vi "Draw.vi"(5 "Angle":dbl, 6 "Scale":sgl=1.0, 7 "Rotation Center":refnum<class "Vector 2D.lvclass">, 8 "error in (no error)":errorcluster, 9 "Destination":refnum<class "Vector 2D.lvclass">, 10 "Texture":refnum<class "Texture.lvclass">, 11 "Renderer":refnum<class "Renderer.lvclass">) -> (0 "error out":errorcluster)   [LabVIEW 2021, in "Renderer.lvclass"]
uses:
  Renderer.lvclass
  Texture/Texture.lvclass
  Vector 2D/Vector 2D.lvclass
  Renderer.lvclass/Renderer.ctl
  LabSDL2/Source/Libraries/LibSDL2 Wrapper/Controls/NULL.ctl
  LabSDL2/Source/Libraries/LibSDL2 Wrapper/LibSDL2.lvlib
  LabSDL2/Source/Libraries/LibSDL2 Wrapper/Controls/Rectangle.ctl
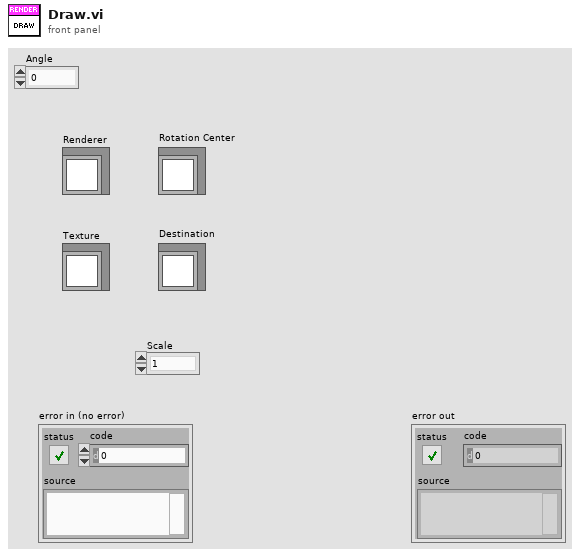
[diagram p1: front panel]
types:
  T1 = typedef "LibSDL2.lvlib/NULL.ctl" = enum32{"NULL"}
  T2 = typedef "LibSDL2.lvlib/Rectangle.ctl" = cluster{"x":i32, "y":i32, "Width":i32, "Height":i32}
  T3 = typedef "SDL2 Utility.lvlib/Point (I32).ctl" = cluster{"x":i32, "y":i32}
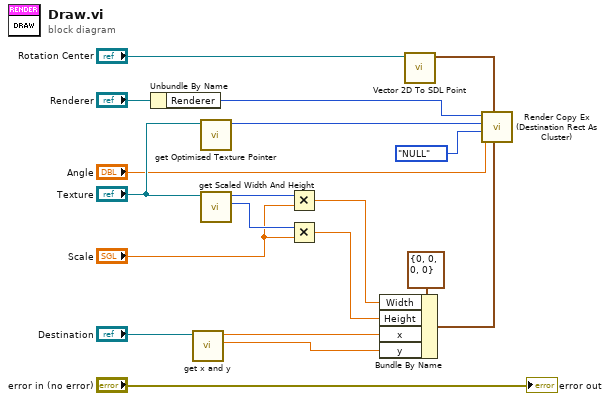
[diagram p0: block diagram]
diagram:
  n1 = Unbundle By Name("Renderer") -> ("Renderer"=w15:u32)
  n2 = call "get x and y.vi"("Vector 2D in"="Destination") -> ("y"=w5:sgl, "x"=w6:sgl)  [unwired: 9 in]
  n3 = call "get Optimised Texture Pointer.vi"("Texture in"="Texture") -> ("Optimised Texture Pointer"=w16:u32)  [unwired: 10 in]
  n4 = call "get Scaled Width And Height.vi"("Texture in"="Texture") -> ("Height"=w10:i32, "Width"=w12:i32)  [unwired: 9 in]
  n5 = Multiply(x=w12, y="Scale") -> (x*y=w11:sgl)
  n6 = Multiply(x=w10, y="Scale") -> (x*y=w9:sgl)
  n7 = Bundle By Name(cluster=T2 {"x"=0, "y"=0, "Width"=0, "Height"=0} ("Destination Rectangle"), "Width"=w11, "Height"=w9, "x"=w6, "y"=w5) -> (w17:T2)
  n8 = call "Vector 2D To SDL Point.vi"("Vector 2D in"="Rotation Center") -> ("Point"=w1:T3)  [unwired: 10 in]
  n9 = call "Render Copy Ex (Destination Rect As Cluster).vi"("Destination Rectangle"=w17, "Point"=w1, "Angle"="Angle", "Source Rectangle Pointer"=NULL."NULL" ("Null"), "Texture Pointer"=w16, "Renderer Pointer"=w15) -> ()  [unwired: 5 in, 1 out]
  "error out" <- "error in (no error)"
